vi "Fire User Event - Stop.vi"(8 "error in (no error)":T1 caption="entrée d'erreur (pas d'erreur)", 11 "Événement utilisateur - Arrêt":refnum<user-event>) -> (0 "error out":T1 caption="sortie d'erreur")   [LabVIEW 2018, in "User Event - Stop.lvlib"]
doc: "Envoyer l'événement Arrêt pour arrêter la boucle de gestion d'événements."
uses:
  User Event - Stop.lvlib
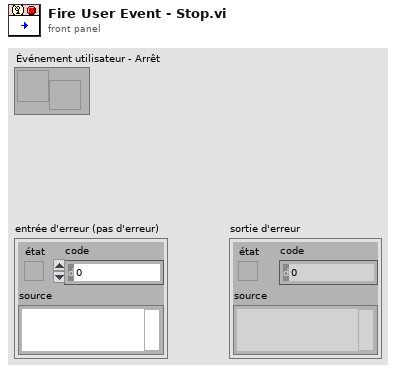
[diagram p1: front panel]
types:
  T1 = cluster{"état":bool, "code":i32, "source":string}
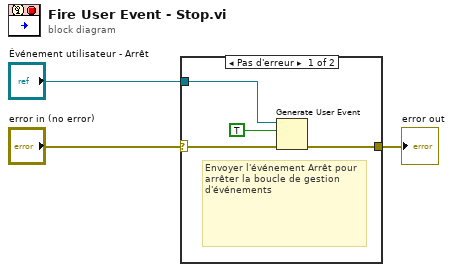
[diagram p0: block diagram]
diagram:
  n1 = case shown="Pas d'erreur" "error in (no error)" {
    selector: "error in (no error)" -> [w4 w8]
    tunnel: [w6 w8] -> w3
    tunnel: "Événement utilisateur - Arrêt" -> [w5 _]
    frame No Error {
      # "Envoyer l'événement Arrêt pour arrêter la boucle de gestion d'événements"
      n2 = Generate User Event(user event=w5, event data cluster=TRUE ("event data"), error in=w4) -> (error out=w6:errorcluster)  [unwired: 1 in, 1 out]
    }
    frame Error {
    }
  }
  "error out" <- w3
